vi "Compare Calls.vi"(8 "error in (no error)":errorcluster, 9 "VI Call 2":refnum<class "VI Call.lvclass">, 10 "VI Call 1":refnum<class "VI Call.lvclass">, 11 "Identical Comparator In":refnum<class "Identical Comparator.lvclass">) -> (0 "error out":errorcluster, 1 "Description":string, 2 "Equal?":bool)   [LabVIEW 2020, in "Identical Comparator.lvclass"]
uses:
  Identical Comparator.lvclass
  Call/VI Call.lvclass
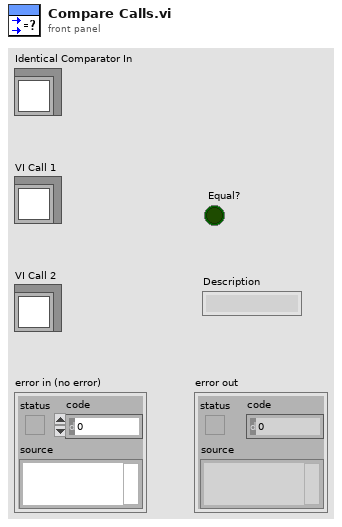
[diagram p1: front panel]
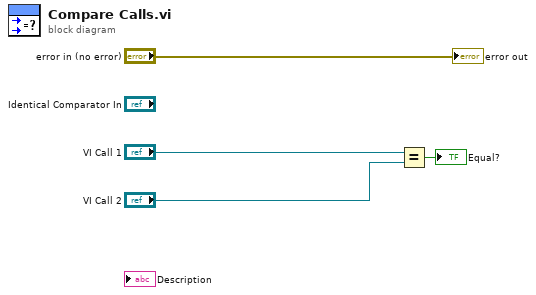
[diagram p0: block diagram]
diagram:
  n1 = Equal?(x="VI Call 1", y="VI Call 2") -> (x = y?=→"Equal?":bool)
  "error out" <- "error in (no error)"
